vi "Rohde & Schwarz VNA Read Power.vi"(6 "Channel":i8=1 min=1 max=99 step=1, 7 "Rohde & Schwarz VNA":T1, 8 "error in (no error)":errorcluster, 11 "VISA Resource Name":refnum<visa-resource-name>) -> (0 "error out":errorcluster, 2 "Source Power, dBm":dbl, 3 "dup VISA Resource Name":refnum<visa-resource-name>)   [LabVIEW 2011]
doc: "This vi sets the power range. Only works on the HP 8753D."
uses:
  TypeDefs/Rohde & Schwarz VNA Instrument Info.ctl
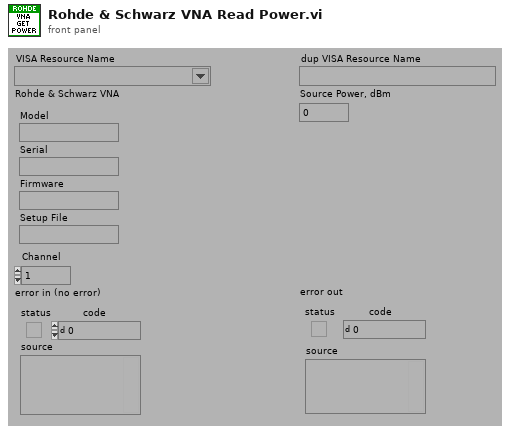
[diagram p1: front panel]
types:
  T1 = typedef "Rohde & Schwarz VNA Instrument Info.ctl" = cluster{"Model":string, "Serial":string, "Firmware":string, "Setup File":string}
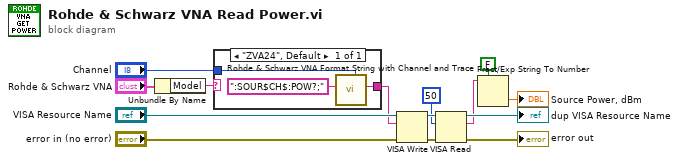
[diagram p0: block diagram]
diagram:
  n1 = Unbundle By Name("Rohde & Schwarz VNA") -> ("Model"=w1:string)
  n2 = case shown="\"ZVA24\", Default" w1 {
    tunnel: [w16] -> w7
    tunnel: "Channel" -> [w15]
    frame "ZVA24", Default {
      n3 = call "Rohde & Schwarz VNA Format String with Channel and Trace.vi"("Trace"=w15, "String"=":SOUR$CH$:POW?;") -> ("String Out"=w16:string)  [unwired: 1 in, 6 out]
    }
  }
  n4 = VISA Write(VISA resource name="VISA Resource Name", write buffer=w7, error in (no error)="error in (no error)") -> (VISA resource name out=w12:refnum<visa-resource-name>, error out=w10:errorcluster)  [unwired: 1 out]
  n5 = VISA Read(VISA resource name=w12, byte count=u32 50, error in (no error)=w10) -> (VISA resource name out=→"dup VISA Resource Name":refnum<visa-resource-name>, read buffer=w5:string, error out=→"error out":errorcluster)  [unwired: 1 out]
  n6 = Fract/Exp String To Number(use system decimal point (T)=FALSE, string=w5) -> (number=→"Source Power, dBm":dbl)  [unwired: 3 out]
